vi "PRAT Main.vi"() -> ()   [LabVIEW 2016]
uses:
  <vilib>/Utility/file.llb/Read From Spreadsheet File (string).vi
panel:
  out "XY Graph":cluster{"DBL":dbl[], "DBL":dbl[]}(graph)
  out "Power Min Value":dbl
  out "Power Max Value":dbl
  out "Power Standard Deviation":dbl format="%0.2f"
  out "Power Mean":dbl format="%0.2f"
  out "Cycle Time (Minutes)":dbl
  out "all rows":string[][](array[string])
  in  "Path":path
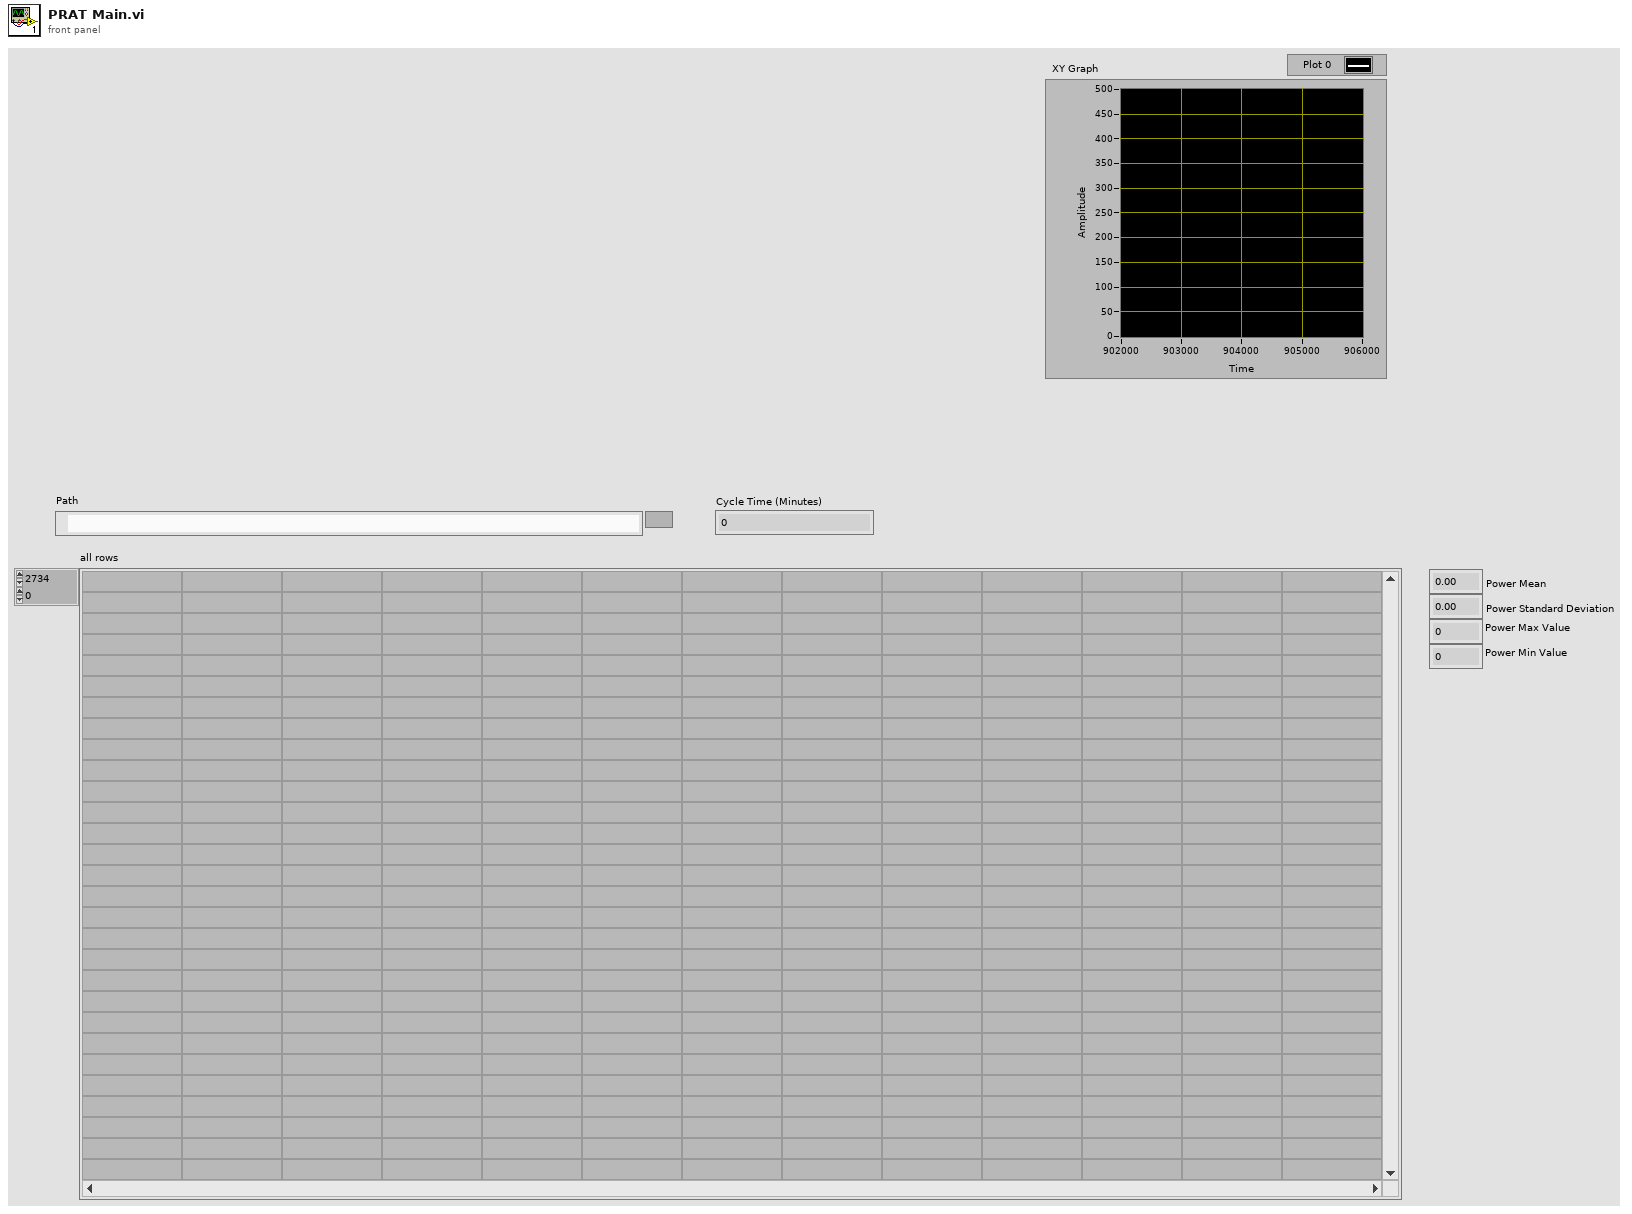
[diagram p1: front panel]
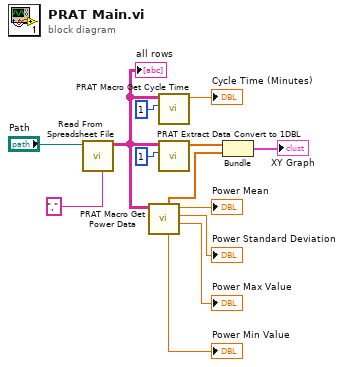
[diagram p0: block diagram]
diagram:
  n1 = call-poly <vilib>:"Read From Spreadsheet File.vi"("delimiter (\\t)"="," ("delimiter (\\t)"), "file path (dialog if empty)"="Path") -> ("all rows"=w8:string[][])  [unwired: 5 in, 4 out]
  "all rows" <- w8
  n2 = call "PRAT Macro Get Power Data.vi"("all rows"=w8) -> ("max value"=→"Power Max Value":dbl, "standard deviation"=→"Power Standard Deviation":dbl, "mean"=→"Power Mean":dbl, "min value"=→"Power Min Value":dbl, "DBL"=w6:dbl[])  [unwired: 5 in, 1 out]
  n3 = call "PRAT Macro Get Cycle Time.vi"("Seconds Column"=1, "Full Cycle Data"=w8) -> ("Cycle Time (Minutes)"=→"Cycle Time (Minutes)":dbl)  [unwired: 8 in, 1 out]
  n4 = call "PRAT Extract Data Convert to 1DBL.vi"("Extract Column"=1, "Full Cycle Data"=w8) -> ("DBL"=w7:dbl[])  [unwired: 8 in, 1 out]
  n5 = Bundle("DBL"=w7, "DBL"=w6) -> (→"XY Graph":cluster{"DBL":dbl[], "DBL":dbl[]})  [unwired: 1 in]
